vi "niFpga wdp fft apply single twid factor.vi"(6 "enable":bool, 8 "data index 1":fxp<+,9,9>, 9 "data index 0":fxp<+,9,9>, 10 "data in 1":T1, 11 "data in 0":T1) -> (2 "data out 1":cluster{"pr":fxp<+/-,25,4>, "pi":fxp<+/-,25,4>}, 3 "data out 0":cluster{"pr":fxp<+/-,25,4>, "pi":fxp<+/-,25,4>})   [LabVIEW 2017]
uses:
  <vilib>/rvi/FXPMathLib/SharedSubVIs/typedef/nifxpmath_BASIC_ImplementationSettings.ctl
  <vilib>/fxp/LVFixedPointQuantizationPolicyTypeDef.ctl
  <vilib>/fxp/LVFixedPointOverflowPolicyTypeDef.ctl
  <vilib>/rvi/Emulation/niFpgaSctlEmulationGetInTimedLoop.vi
  <vilib>/Utility/error.llb/Clear Errors.vi
  <vilib>/rvi/DataTransferAndStorage/Container/Common/niFpgaContainerGetUniqueNameForEmu.vi
  <vilib>/rvi/DataTransferAndStorage/Container/Common/niFpgaContainerSetEmuInfo.vi
  <vilib>/rvi/eio/common/nirviEmuReportErrorAndStop.vi
  <vilib>/rvi/DataTransferAndStorage/Container/Common/niFpgaContainerExecOnDevCompGetState.vi
  <vilib>/rvi/Emulation/niFpgaEmulationIsFPGAContextNoSignature.vi
  <vilib>/rvi/Emulation/niFpgaProcessEmulError.vi
  <vilib>/rvi/errors/nirviReportUnexpectedCaseInternalError (U32).vi
  <vilib>/rvi/Memory/Memory_Emulation/niFpgaMemoryEmulationCacheClearOnFirstRun.vi
  <vilib>/rvi/Memory/Memory_Emulation/nirvimemoryEmulationManagerCache_MakeExclusive.vi
  <vilib>/rvi/Memory/Memory_Emulation/niFpgaMemoryEmulationValidateCache.vi
  <vilib>/rvi/Memory/Memory_Emulation/nirvimemoryEmulationManagerCache_InsertValue.vi
  <vilib>/rvi/Memory/Memory_Emulation/nirvimemoryEmulationManagerCache_ReleaseExclusive.vi
  <vilib>/rvi/Memory/Memory_Emulation/nirvimemoryEmulationManagerCache_GetValue.vi
  <vilib>/rvi/Memory/Memory_Emulation/nirvimemoryEmulationManagerCache_SetValue.vi
  <vilib>/rvi/Emulation/niFpgaSctlEmulationResourceMgr.vi
  <vilib>/rvi/ClientSDK/Core/DevComputerLib/Private/FourWireProtocol(cint64).vi
  <vilib>/rvi/FXPMathLib/basic elements/FxpDiscreteDelay/XNode/nifxpmath_DiscreteDelay.xnode
  <vilib>/rvi/LocalResourceManager/LocalResourceManager.xnode
  <vilib>/rvi/DataTransferAndStorage/Container/XNode/niFpgaContainer.xnode
  <vilib>/rvi/Memory/Memory_Emulation/niFpgaMemoryEmulationRefIn.vi
  <vilib>/rvi/FXPMathLib/FxpMultComplex/XNode/niFpgaMultComplex.xnode
  <vilib>/rvi/ClientSDK/Core/DevComputerLib/niFpgaDevCompUtilities.lvlib
types:
  T1 = cluster{"data re":fxp<+/-,8,1>, "data im":fxp<+/-,8,1>}
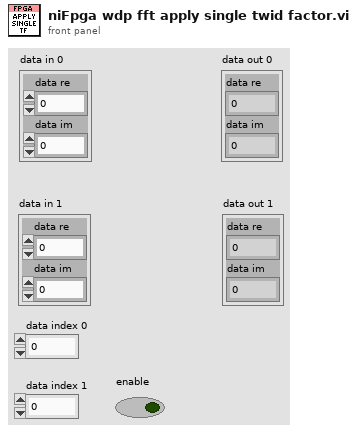
[diagram p1: front panel]
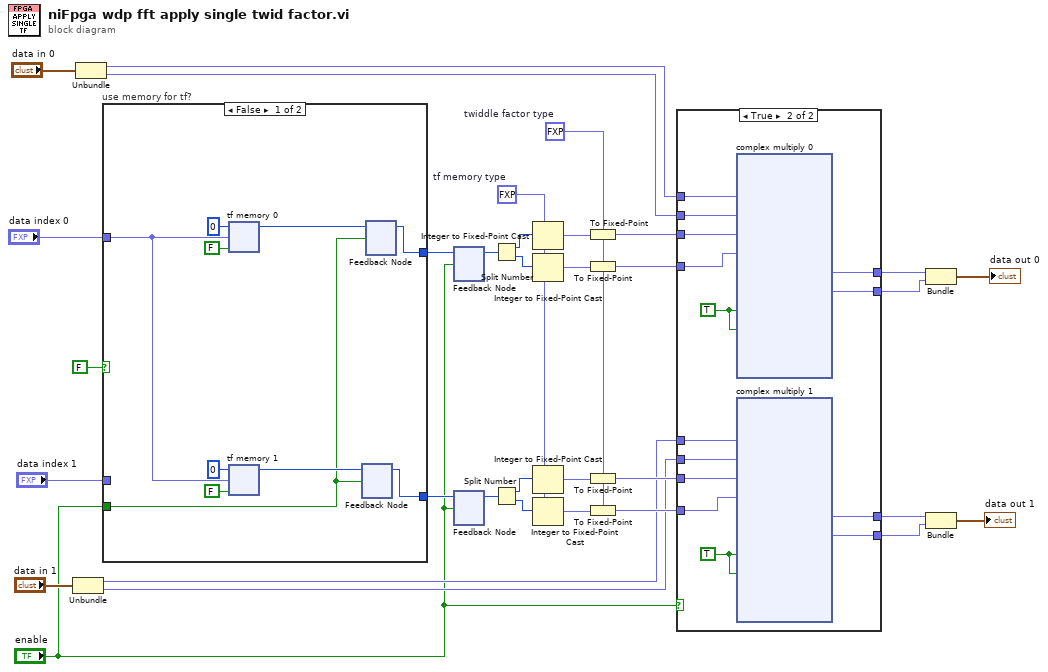
[diagram p0: block diagram]
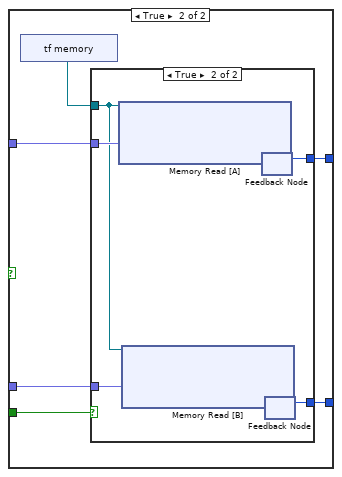
[diagram p2: hidden frame]
diagram:
  w24 = fxp<+/-,16,2> 0.0  # twiddle factor type
  w34 = fxp<+/-,16,2> 0.0  # tf memory type
  n1 = Unbundle("data in 1") -> ("data re"=w11:fxp<+/-,8,1>, "data im"=w10:fxp<+/-,8,1>)
  n2 = Unbundle("data in 0") -> ("data re"=w9:fxp<+/-,8,1>, "data im"=w12:fxp<+/-,8,1>)
  n3 = case "use memory for tf?" shown="False" FALSE {
    tunnel: [w37 w50] -> w22
    tunnel: [w41 w49] -> w21
    tunnel: "data index 0" -> [w35 w48]
    tunnel: "data index 1" -> [_ w47]
    tunnel: "enable" -> [w36 w46]
    frame False {
      n4 = xnode "tf memory 0"("D"=u32 0, "n-1[0..15]"=w35, "enable"=FALSE) -> ("Q"=w44:u32)
      n5 = xnode "tf memory 1"("D"=u32 0, "n-1[0..15]"=w35, "enable"=FALSE) -> ("Q"=w38:u32)
      n6 = feedback #1() -> (w37:u32)  [unwired: 1 in]
      n7 = feedback-in #1(w38, w36) -> ()
      n8 = feedback #2() -> (w41:u32)  [unwired: 1 in]
      n9 = feedback-in #2(w44, w36) -> ()
    }
    frame True {
      n10 = xnode "tf memory"() -> ("Memory Out"=w45:refnum<k21>)
      n11 = case shown="True" w46 {
        tunnel: w48 -> [_ w57]
        tunnel: w47 -> [_ w54]
        tunnel: [_ w53] -> w49
        tunnel: [_ w52] -> w50
        tunnel: w45 -> [_ w51]
        frame False {
        }
        frame True {
          n12 = xnode ("Memory Read [A]")("Address A"=w57, "Memory In"=w51) -> ("Data A"=w56:u32)  [unwired: 1 out]
          n13 = xnode ("Memory Read [B]")("Address B"=w54, "Memory In"=w51) -> ("Data B"=w55:u32)  [unwired: 1 out]
          n14 = feedback #3() -> (w53:u32)  [unwired: 1 in]
          n15 = feedback-in #3(w56) -> ()
          n16 = feedback #4() -> (w52:u32)  [unwired: 1 in]
          n17 = feedback-in #4(w55) -> ()
        }
      }
    }
  }
  n18 = feedback #5() -> (w28:u32)  [unwired: 1 in]
  n19 = feedback-in #5(w21, "enable") -> ()
  n20 = feedback #6() -> (w33:u32)  [unwired: 1 in]
  n21 = feedback-in #6(w22, "enable") -> ()
  n22 = Split Number(x=w28) -> (hi(x)=w27:u16, lo(x)=w26:u16)
  n23 = Split Number(x=w33) -> (hi(x)=w29:u16, lo(x)=w30:u16)
  n24 = Integer to Fixed-Point Cast(fixed-point type=w34, integer=w27) -> (fixed-point=w25:fxp<+/-,16,2>)
  n25 = Integer to Fixed-Point Cast(fixed-point type=w34, integer=w26) -> (fixed-point=w23:fxp<+/-,16,2>)
  n26 = Integer to Fixed-Point Cast(fixed-point type=w34, integer=w29) -> (fixed-point=w31:fxp<+/-,16,2>)
  n27 = Integer to Fixed-Point Cast(fixed-point type=w34, integer=w30) -> (fixed-point=w32:fxp<+/-,16,2>)
  n28 = To Fixed-Point(fixed-point type=w24, number=w25) -> (fixed-point=w18:fxp<+/-,16,2>)
  n29 = To Fixed-Point(fixed-point type=w18, number=w23) -> (fixed-point=w17:fxp<+/-,16,2>)
  n30 = To Fixed-Point(fixed-point type=w18, number=w31) -> (fixed-point=w16:fxp<+/-,16,2>)
  n31 = To Fixed-Point(fixed-point type=w16, number=w32) -> (fixed-point=w15:fxp<+/-,16,2>)
  n32 = case shown="True" "enable" {
    tunnel: w18 -> [_ w69]
    tunnel: w17 -> [_ w68]
    tunnel: w16 -> [_ w67]
    tunnel: w15 -> [_ w66]
    tunnel: w9 -> [_ w65]
    tunnel: w12 -> [_ w64]
    tunnel: w11 -> [_ w63]
    tunnel: w10 -> [_ w62]
    tunnel: [_ w61] -> w6
    tunnel: [_ w60] -> w5
    tunnel: [_ w59] -> w4
    tunnel: [_ w58] -> w3
    frame False {
    }
    frame True {
      w70 = TRUE ("enable")
      w71 = TRUE ("enable")
      n33 = xnode "complex multiply 0"("xr"=w65, "xi"=w64, "yr"=w69, "yi"=w68, "input valid"=w71, "ready for output (T)"=w71) -> ("pr"=w61:fxp<+/-,25,4>, "pi"=w60:fxp<+/-,25,4>)  [unwired: 2 out]
      n34 = xnode "complex multiply 1"("xr"=w63, "xi"=w62, "yr"=w67, "yi"=w66, "input valid"=w70, "ready for output (T)"=w70) -> ("pr"=w59:fxp<+/-,25,4>, "pi"=w58:fxp<+/-,25,4>)  [unwired: 2 out]
    }
  }
  n35 = Bundle("pr"=w6, "pi"=w5) -> (→"data out 0":cluster{"pr":fxp<+/-,25,4>, "pi":fxp<+/-,25,4>})  [unwired: 1 in]
  n36 = Bundle("pr"=w4, "pi"=w3) -> (→"data out 1":cluster{"pr":fxp<+/-,25,4>, "pi":fxp<+/-,25,4>})  [unwired: 1 in]
